vi "e_diff_test.vi"() -> ()   [LabVIEW 2013]
panel:
  out "Array 3":dbl[](array[numeric])
  out "Waveform Graph":dbl[][](graph)
  out "Array 2":fxp<+/-,32,4>[](array[numeric])
  out "Array":bool[](array[boolean])
  out "Numeric":i32
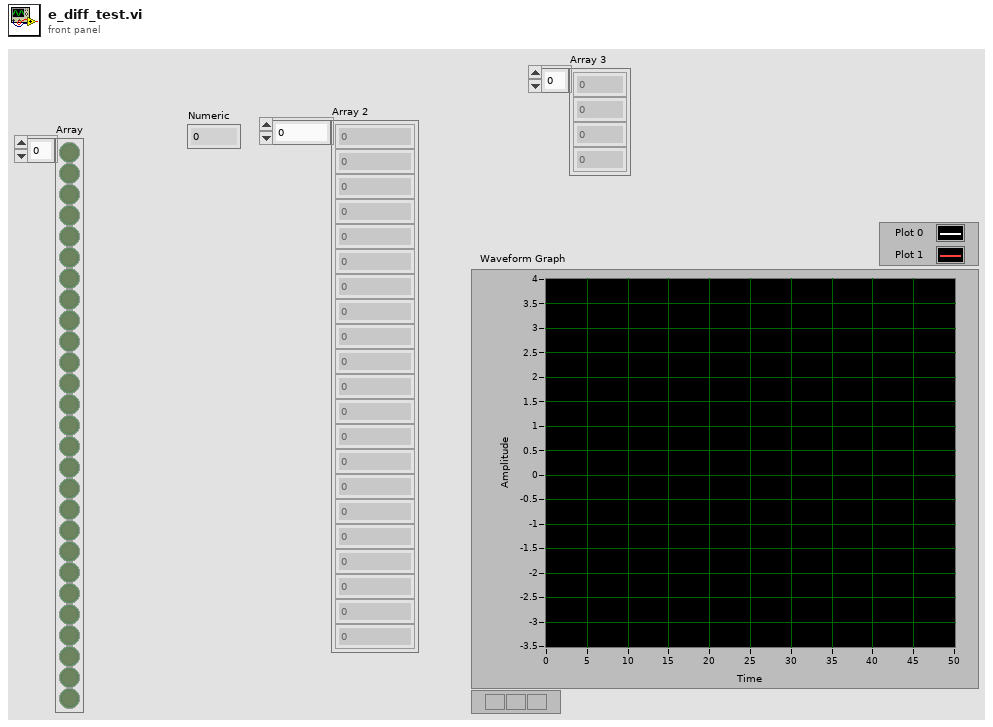
[diagram p1: front panel]
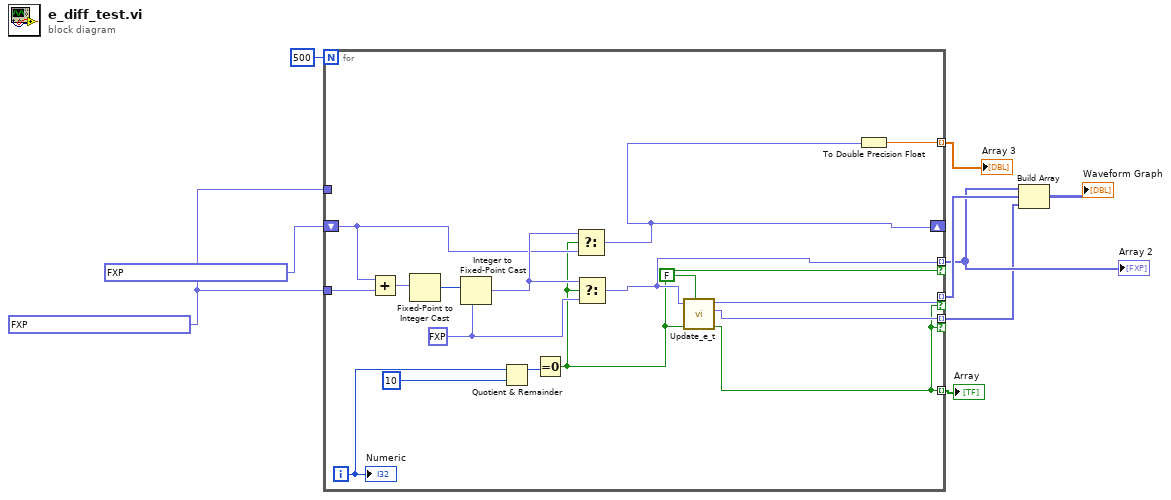
[diagram p0: block diagram]
diagram:
  w6 = fxp<+/-,31,3> -0.14999999850988388 ("y")
  n1 = for {
    N: 500 -> [_]
    tunnel: [w15] -> w2 mode=indexing if=w12
    tunnel: w6 -> [w26]
    tunnel: [w22] -> w7 mode=indexing
    shift-right: [w16] -> _
    shift-left: fxp<+/-,31,3> 3.9999999962747097 ("wrap_max") -> [w17]
    tunnel: w6 -> [_]
    tunnel: [w11] -> w5 mode=indexing
    tunnel: [w14] -> w4 mode=indexing if=w11
    tunnel: [w13] -> w1 mode=indexing if=w11
    i -> [w25]
    w19 = fxp<+/-,32,4> 0.0 ("f")
    n2 = Add(x=w17, y=w26) -> (x+y=w21:fxp<+/-,33,5>)
    n3 = Fixed-Point to Integer Cast(1:w21) -> (0:w20:i64)
    n4 = Integer to Fixed-Point Cast(fixed-point type=w19, integer=w20) -> (fixed-point=w18:fxp<+/-,32,4>)
    n5 = Quotient & Remainder(x=w25, y=10) -> (x-y*floor(x/y)=w23:i32)  [unwired: 1 out]
    n6 = Equal To 0?(x=w23) -> (x = 0?=w12:bool)
    n7 = Select(t=w18, s=w12, f=w17) -> (s? t:f=w16:fxp<+/-,32,4>)
    n8 = Select(t=w18, s=w12, f=w19) -> (s? t:f=w15:fxp<+/-,32,4>)
    n9 = call "Update_e_t.vi"("Rest"=FALSE, "input valid"=w12, "e(t)"=w15) -> ("output valid"=w11:bool, "e(t-1)-e(t-2)"=w13:fxp<+/-,32,4>, "e(t)-e(t-1)"=w14:fxp<+/-,32,4>)  [unwired: 6 in]
    n10 = To Double Precision Float(number=w16) -> (double precision float=w22:dbl)
    "Numeric" <- w25
  }
  "Array" <- w5
  "Array 2" <- w2
  "Array 3" <- w7
  n11 = Build Array(w2, w4, w1) -> (→"Waveform Graph":fxp<+/-,32,4>[][])
